vi "15.vi"() -> ()   [LabVIEW 2021]
uses:
  <vilib>/gmath/NI_Gmath.lvlib
panel:
  out "SW Lattice Paths":dbl
  in  "Number of Columns":i32=20
  in  "Number of Rows":i32=20
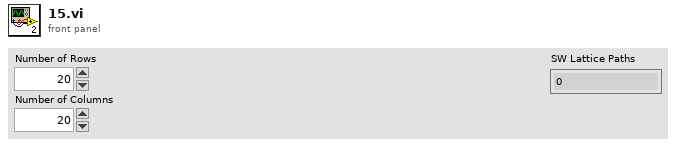
[diagram p1: front panel]
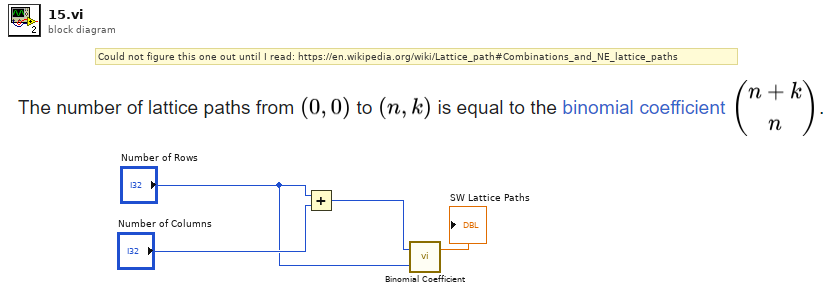
[diagram p0: block diagram]
diagram:
  # "Could not figure this one out until I read: https://en.wikipedia.org/wiki/Lattice_path#Combinations_and_NE_lattice_paths"
  n1 = Add(x="Number of Rows", y="Number of Columns") -> (x+y=w3:i32)
  n2 = call <vilib>:"Binomial Coefficient.vi"("k"="Number of Rows", "n"=w3) -> ("binomial coefficient (n,k)"=→"SW Lattice Paths":dbl)  [unwired: 1 out]
